vi "InitializeRoot.vi"(8 "error in (no error)":errorcluster, 10 "InitRoot":T1, 11 "xceRootNode in":refnum<class "xceRootNode.lvclass">) -> (0 "error out":errorcluster, 3 "RootNode*":refnum<data-value>)   [LabVIEW 2013, in "xceRootNode.lvclass"]
doc: "Initializes a Root based on common inputs to the root node, i.e. a tree control reference, glyph directory, and top-level menu reference."
uses:
  xceRootNode.lvclass
  RootInit.ctl
  xceRootNode.lvclass/xceRootNode.ctl
  xceNode/xceNode.lvclass
  xceDataNode/xceDataNode.lvclass
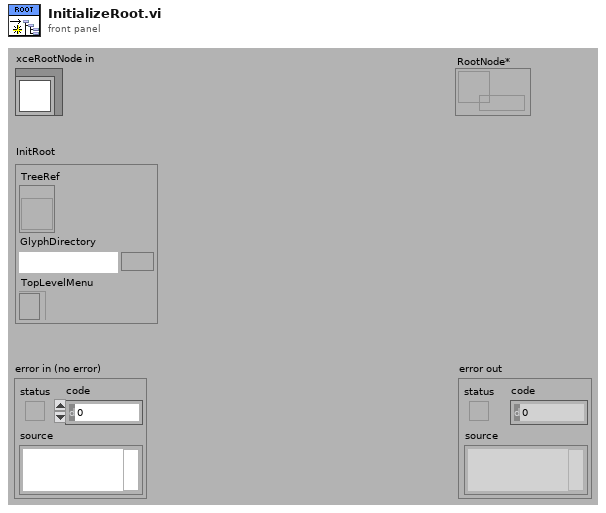
[diagram p1: front panel]
types:
  T1 = typedef "xceRootNode.lvclass/RootInit.ctl" = cluster{"TreeRef":refnum<vi>, "GlyphDirectory":path, "TopLevelMenu":refnum<k9>}
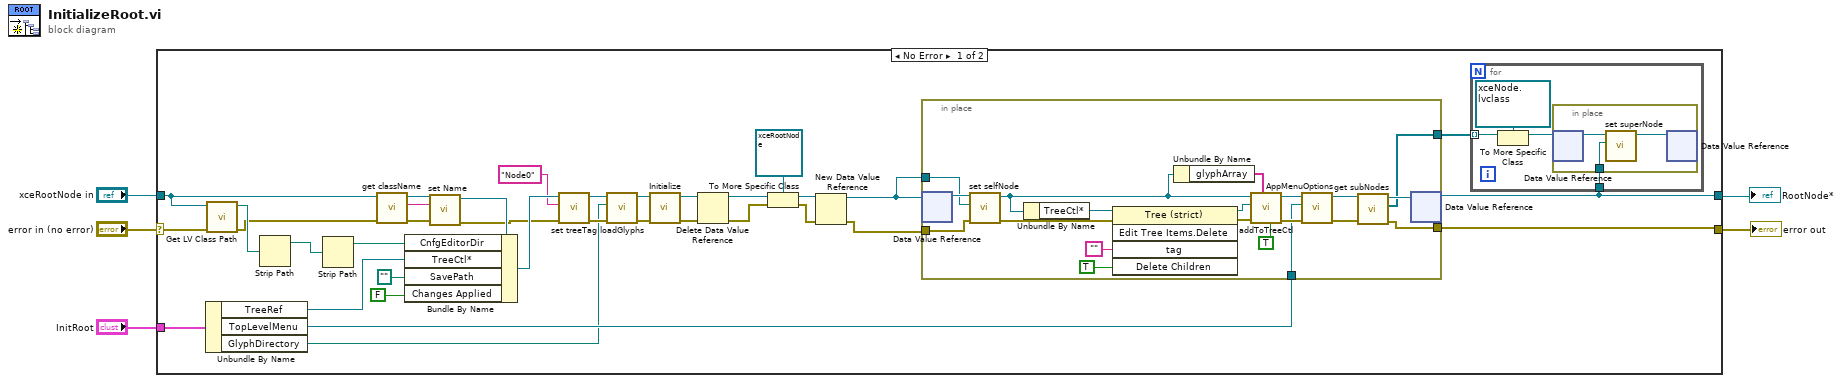
[diagram p0: block diagram]
diagram:
  n1 = case shown="No Error" "error in (no error)" {
    selector: "error in (no error)" -> [w25 w68]
    tunnel: [w22 w68] -> w4
    tunnel: [w18 _] -> w2
    tunnel: "xceRootNode in" -> [w12 _]
    tunnel: "InitRoot" -> [w37 _]
    frame No Error {
      n2 = Unbundle By Name(w37) -> ("TreeRef"=w36:refnum<vi>, "TopLevelMenu"=w20:refnum<k9>, "GlyphDirectory"=w13:path)
      n3 = call <vilib>:"Get LV Class Path.vi"("error in (no error)"=w25, "object"=w12) -> ("error out"=w11:errorcluster, "class path"=w40:path)  [unwired: 8 in]
      n4 = Strip Path(path=w40) -> (stripped path=w39:path)  [unwired: 1 out]
      n5 = Strip Path(path=w39) -> (stripped path=w38:path)  [unwired: 1 out]
      n6 = call "get className.vi"("error in (no error)"=w11, "xceNode in"=w12) -> ("error out"=w9:errorcluster, "Class name"=w8:string, "xceNode out"=w10:refnum<class "xceRootNode.lvclass">)  [unwired: 7 in]
      n7 = call "set Name.vi"("error in (no error)"=w9, "Name"=w8, "xceDataNode in"=w10) -> ("error out"=w6:errorcluster, "xceDataNode out"=w7:refnum<class "xceRootNode.lvclass">)  [unwired: 7 in]
      n8 = Bundle By Name(cluster=w7, "CnfgEditorDir"=w38, "TreeCtl*"=w36, "SavePath"=path "", "Changes Applied"=FALSE) -> (w24:refnum<class "xceRootNode.lvclass">)
      n9 = call "set treeTag.vi"("error in (no error)"=w6, "treeTag"="Node0", "xceNode in"=w24) -> ("error out"=w17:errorcluster, "xceNode out"=w16:refnum<class "xceRootNode.lvclass">)  [unwired: 7 in]
      n10 = call "loadGlyphs.vi"("error in (no error)"=w17, "Glyph Dir"=w13, "xceRootNode in"=w16) -> ("error out"=w14:errorcluster, "xceRootNode out"=w15:refnum<class "xceRootNode.lvclass">)  [unwired: 7 in]
      n11 = call-dynamic "Initialize.vi"("error in"=w14, "xceRootNode in"=w15) -> ("error out"=w26:errorcluster, "Node*"=w33:refnum<data-value>)  [unwired: 8 in]
      n12 = Delete Data Value Reference(data value reference=w33, error in=w26) -> (data value=w31:refnum<class "xceNode.lvclass">, error out=w32:errorcluster)
      n13 = To More Specific Class(target class=refnum<class "xceRootNode.lvclass"> refnum ("output cluster"), reference=w31, error in=w32) -> (specific class reference=w28:refnum<class "xceRootNode.lvclass">, error out=w29:errorcluster)
      n14 = New Data Value Reference(data value=w28, error in=w29) -> (data value reference=w21:refnum<data-value>, error out=w27:errorcluster)
      n15 = in-place {
        in-place-border: w27 -> [w66]
        in-place-border: [w52] -> w22
        in-place-border: w21 -> [w65]
        in-place-border: w20 -> [w57]
        in-place-border: [w51] -> w19
        n16 = in-place-dvr #1(w21) -> (w67:refnum<class "xceRootNode.lvclass">)  [unwired: 1 out]
        n17 = call "set selfNode.vi"("error in (no error)"=w66, "selfNode*"=w65, "xceNode in"=w67) -> ("error out"=w56:errorcluster, "xceNode out"=w50:refnum<class "xceRootNode.lvclass">)  [unwired: 7 in]
        n18 = Unbundle By Name(w50) -> ("TreeCtl*"=w64:refnum<vi>)
        n19 = invoke class="Tree (strict)" method="Edit Tree Items.Delete"(reference=w64, error in=w56, "tag"="", "Delete Children"=TRUE ("Delete Children?")) -> (reference out=w62:refnum<vi>, error out=w61:errorcluster)  [unwired: 1 in, 3 out]
        n20 = Unbundle By Name(w50) -> ("glyphArray"=w49:string[])
        n21 = call "addToTreeCtl.vi"("AppendToEnd"=TRUE, "glyphArray"=w49, "error in (no error)"=w61, "TreeCtl*"=w62, "xceDataNode in"=w50) -> ("error out"=w59:errorcluster, "xceDataNode out"=w58:refnum<class "xceRootNode.lvclass">)  [unwired: 5 in]
        n22 = call-dynamic "AppMenuOptions.vi"("error in (no error)"=w59, "appMenu* in"=w57, "xceRootNode in"=w58) -> ("error out"=w53:errorcluster, "xceRootNode out"=w55:refnum<class "xceRootNode.lvclass">)  [unwired: 6 in, 1 out]
        n23 = call "get subNodes.vi"("error in (no error)"=w53, "xceNode in"=w55) -> ("error out"=w52:errorcluster, "subNodes[]*"=w51:refnum<data-value>[], "xceNode out"=w54:refnum<class "xceRootNode.lvclass">)  [unwired: 7 in]
        n24 = in-place-dvr #1(w54) -> (w18:refnum<data-value>)  [unwired: 1 out]
      }
      n25 = for {
        tunnel: w19 -> [w44] mode=indexing
        tunnel: w18 -> [w41]
        n26 = To More Specific Class(target class=refnum<data-value> refnum ("data value reference"), reference=w44) -> (specific class reference=w42:refnum<data-value>)  [unwired: 1 in, 1 out]
        n27 = in-place {
          in-place-border: w41 -> [w46]
          n28 = in-place-dvr #2(w42) -> (w47:refnum<class "xceNode.lvclass">)  [unwired: 1 out]
          n29 = call "set superNode.vi"("superNode*"=w46, "xceNode in"=w47) -> ("xceNode out"=w45:refnum<class "xceNode.lvclass">)  [unwired: 8 in, 1 out]
          n30 = in-place-dvr #2(w45) -> ()  [unwired: 2 out]
        }
      }
    }
    frame Error {
    }
  }
  "error out" <- w4
  "RootNode*" <- w2
